vi "Pet Feeder.vi"() -> ()   [LabVIEW 2019, in "Pet Feeder.lvlib"]
uses:
  Pet Feeder.lvlib
  Types/app_event.ctl
  Types/state_machine_event.ctl
  Controls/Feeder Program.ctl
  Types/internal_state_data.ctl
  Types/state.ctl
panel:
  in  "clear last?":bool
  out "state":T1
  out "internal state data":T2 {"last dispense time" format="%<%H:%M:%S>t"; "clock time" format="%<%H:%M:%S>t"}
  in  "stop":bool
  in  "hopper level":i32=16
  out "hopper empty":bool
  out "hopper low":bool
  in  "set hopper":bool
  in  "set simulated time":bool
  in  "simulated time":string(combo)="1:00:00 PM"
  out "timer (s)":dbl format="%1.1g"
  out "remaining servings":i32(slide) scale=0.0..100.0
  in  "decrement servings":bool
  in  "increment servings":bool
  in  "program mode":string(combo)="none"
  in  "decrement minute":bool
  in  "increment minute":bool
  in  "decrement hour":bool
  in  "increment hour":bool
  out "current time":string
  out "schedule":T3[](array[typedef])
  in  "dispense serving":bool
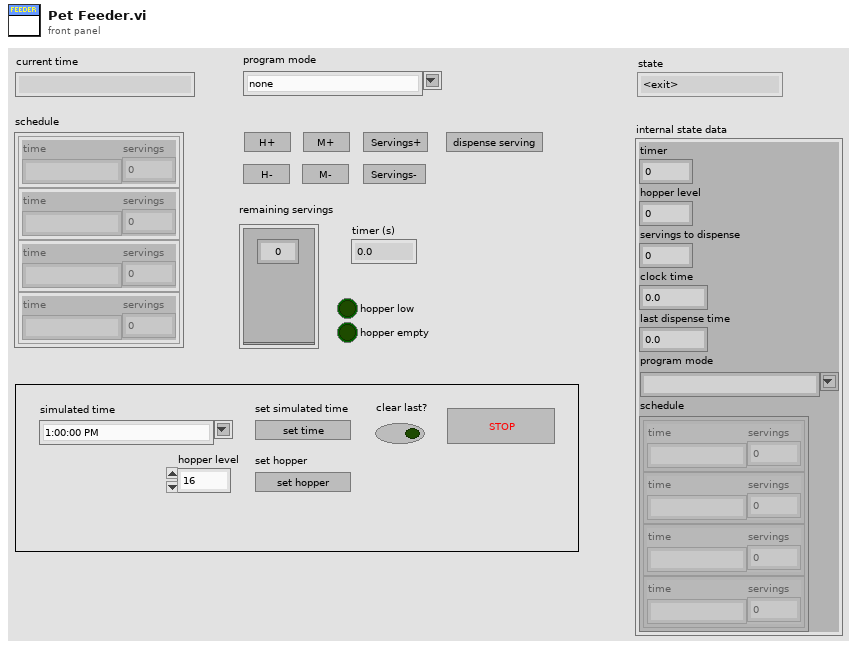
[diagram p1: front panel]
types:
  T1 = typedef "Pet Feeder.lvlib/state.ctl" = enum16{"<exit>", "<entry>", "idle", "dispensing"}
  T2 = typedef "Pet Feeder.lvlib/internal_state_data.ctl" = cluster{"timer":dbl, "hopper level":i32, "servings to dispense":i32, "clock time":dbl, "last dispense time":dbl, "program mode":string, "schedule":T3[]}
  T3 = typedef "Pet Feeder.lvlib/Feeder Program.ctl" = cluster{"time":string, "servings":i32}
  T4 = typedef "Pet Feeder.lvlib/state_machine_event.ctl" = cluster{"event":enum16{"button press", "timeout"}, "data":string}
  T5 = typedef "Pet Feeder.lvlib/app_event.ctl" = enum16{"Initialize", "Shutdown", "Exit"}
  T6 = cluster{"event":enum16{"button press", "timeout"}, "data":string}
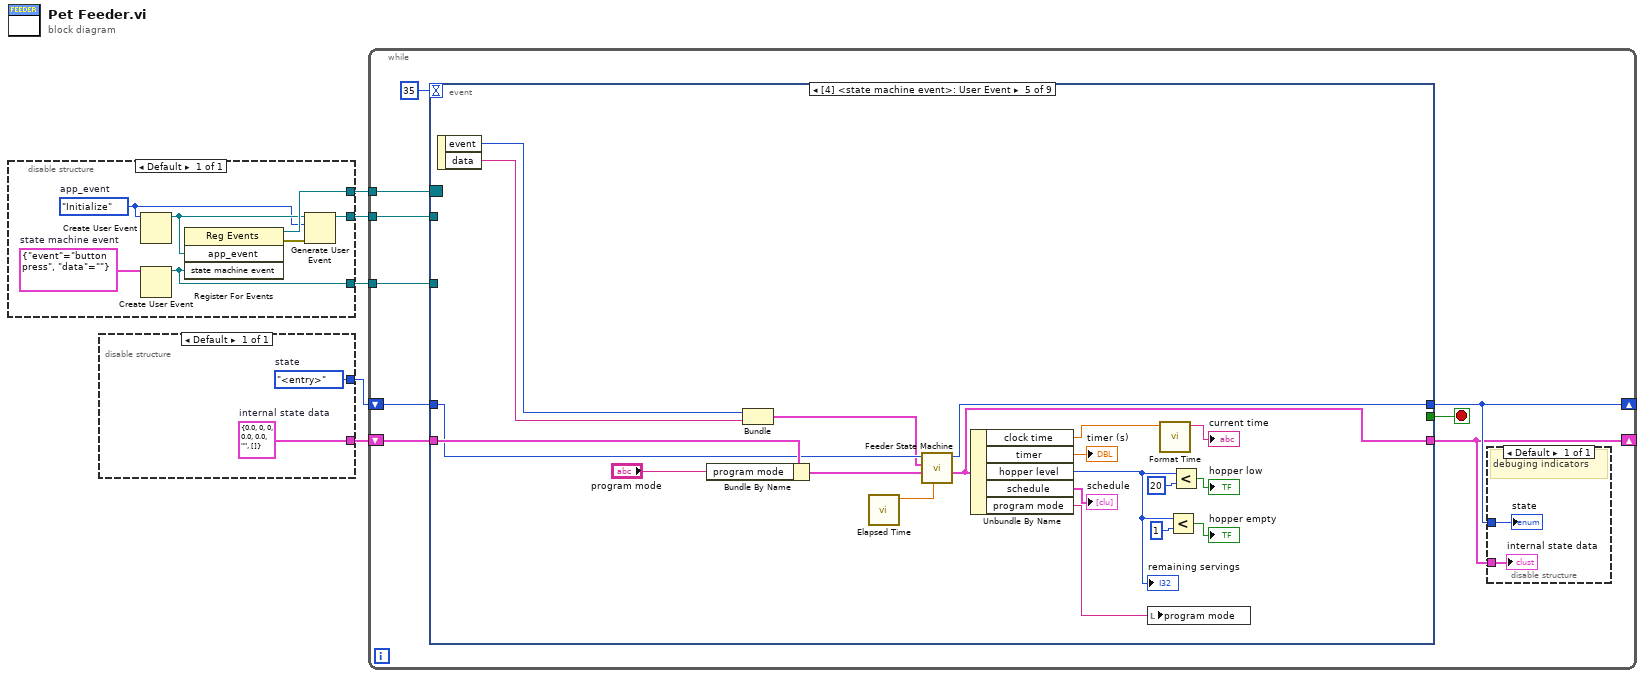
[diagram p0: block diagram]
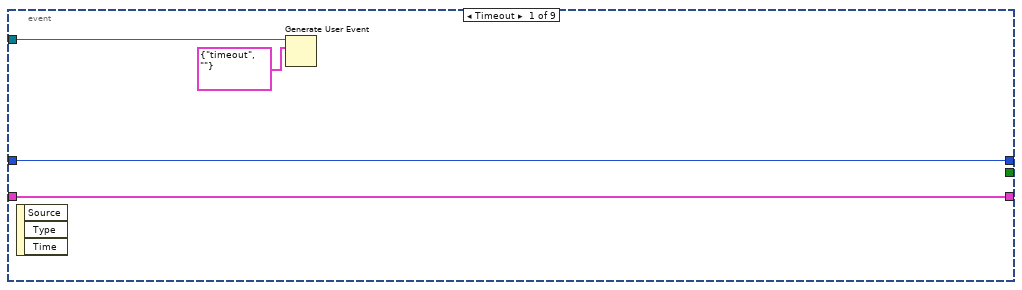
[diagram p2: hidden frame]
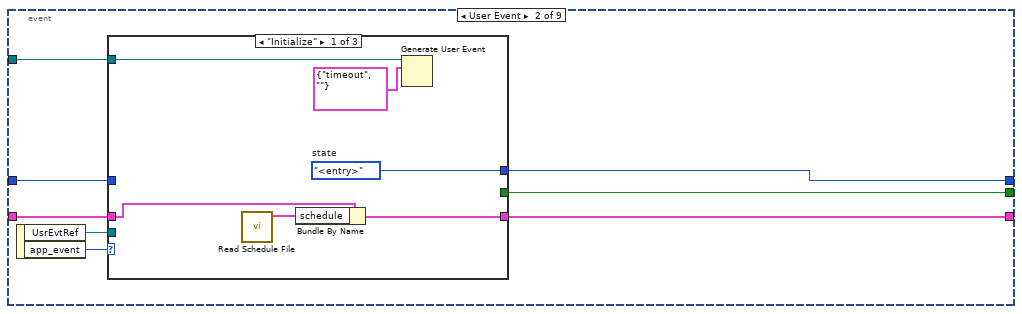
[diagram p3: hidden frame]
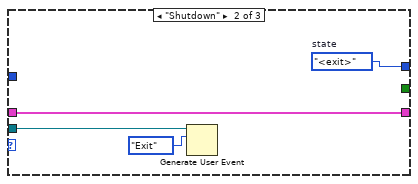
[diagram p4: hidden frame]
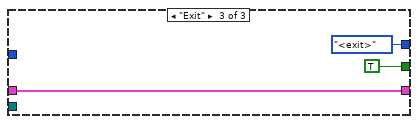
[diagram p5: hidden frame]
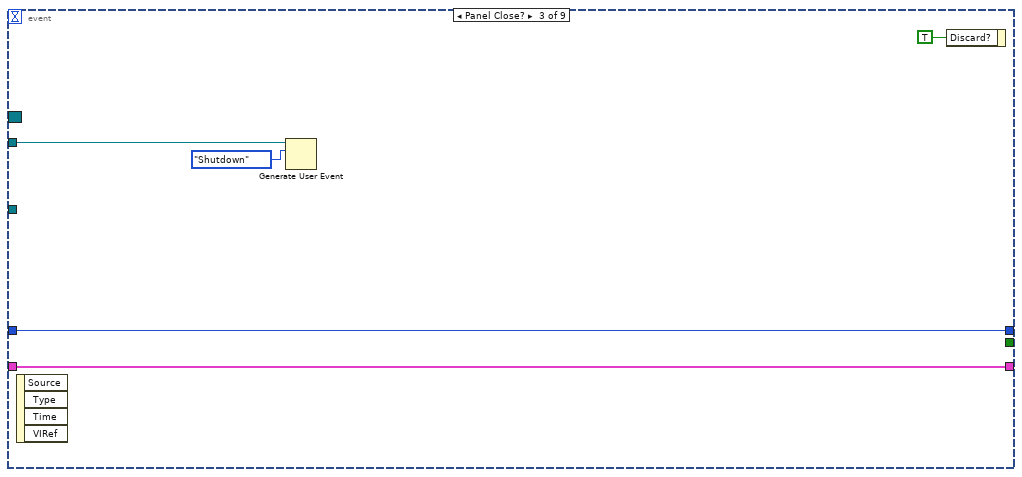
[diagram p6: hidden frame]
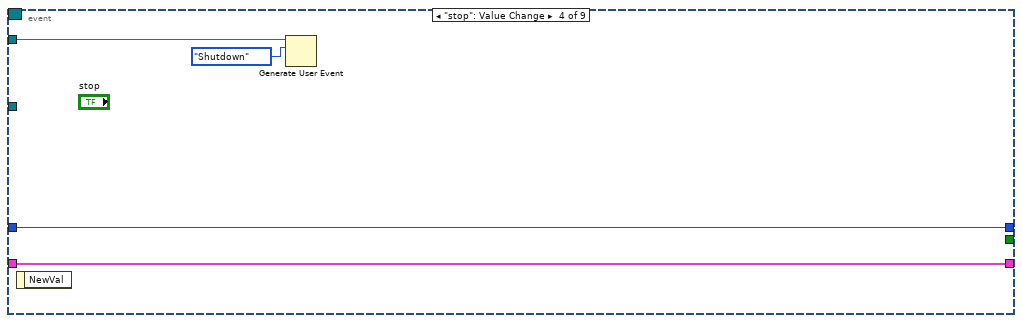
[diagram p7: hidden frame]
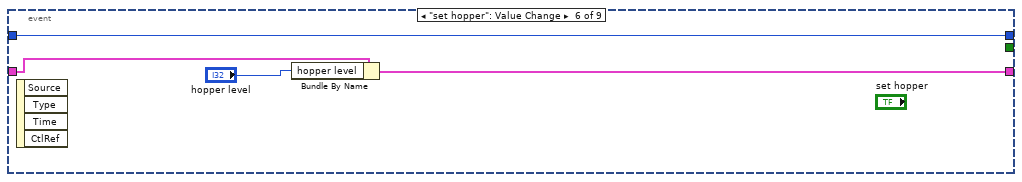
[diagram p8: hidden frame]
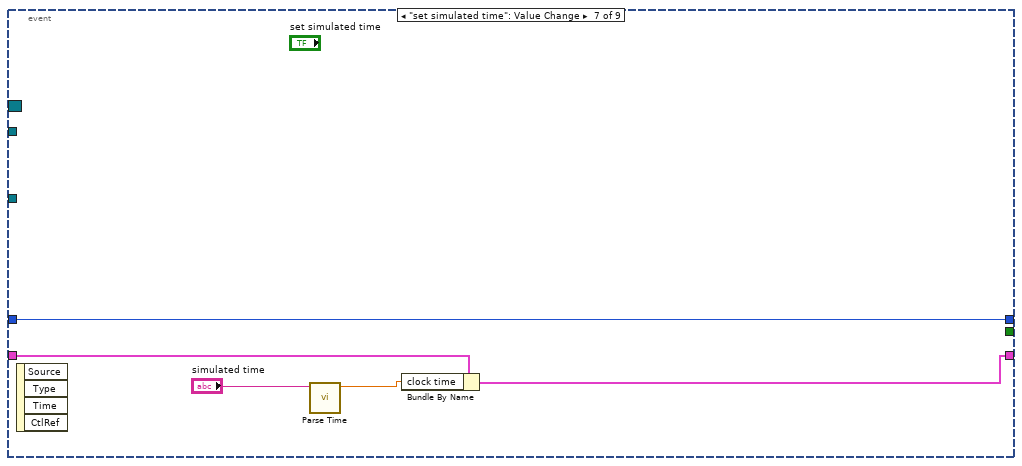
[diagram p9: hidden frame]
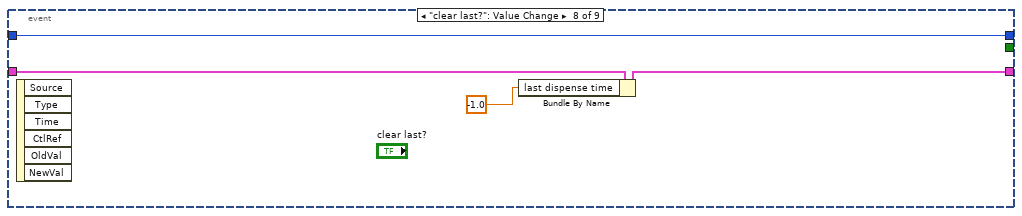
[diagram p10: hidden frame]
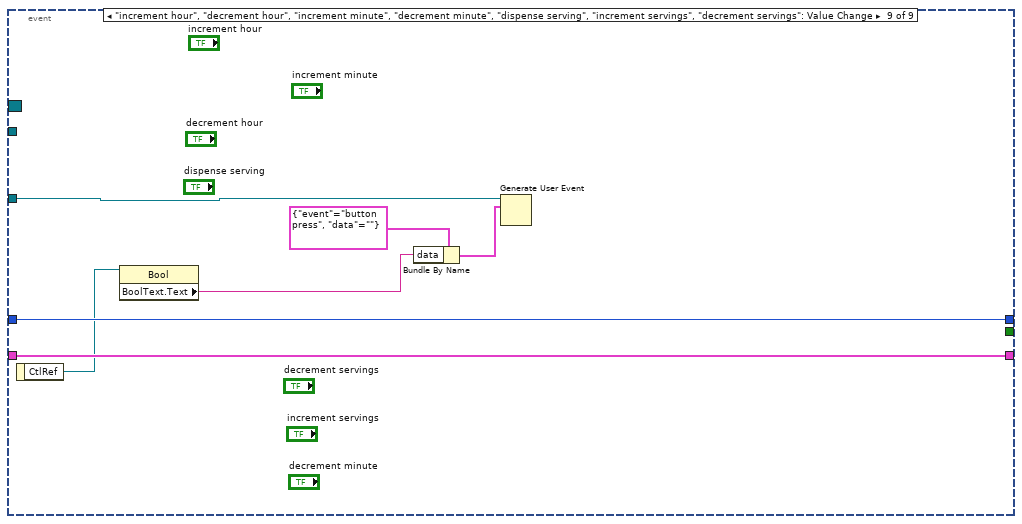
[diagram p11: hidden frame]
diagram:
  n1 = disable-structure shown="Default" {
    disable-tunnel: [w12] -> w5
    disable-tunnel: [w7] -> w4
    disable-tunnel: [w6] -> w3
    frame Enabled {
      w11 = T4 {"event"=enum."button press", "data"=""}  # state machine event
      w8 = app_event."Initialize"  # app_event
      n2 = Create User Event(user event datatype=w8) -> (user event=w10:refnum<user-event>)  [unwired: 1 in, 1 out]
      n3 = Create User Event(user event datatype=w11) -> (user event=w6:refnum<user-event>)  [unwired: 1 in, 1 out]
      n4 = register-events(w10, w6) -> (reference out=w12:refnum<event-registration>, error out=w9:errorcluster)  [unwired: 2 in]
      n5 = Generate User Event(user event=w10, event data cluster=w8, error in=w9) -> (user event out=w7:refnum<user-event>)  [unwired: 1 in, 1 out]
    }
  }
  n6 = disable-structure shown="Default" {
    disable-tunnel: [w14] -> w2
    disable-tunnel: [w13] -> w1
    frame Enabled {
      w14 = state."<entry>"  # state
      w13 = T2 {"timer"=0.0, "hopper level"=0, "servings to dispense"=0, "clock time"=0.0, "last dispense time"=0.0, "program mode"="", "schedule"=[]}  # internal state data
    }
  }
  n7 = while {
    tunnel: w5 -> [w23]
    tunnel: w4 -> [w15]
    tunnel: w3 -> [w18]
    shift-right: [w21] -> _
    shift-left: w2 -> [w22]
    shift-right: [w20] -> _
    shift-left: w1 -> [w19]
    stop <- w17 stop-if-true
    n8 = event shown="[4] <state machine event>: User Event" {
      selector: w23 -> [_ _ _ _ _ _ _ _ _]
      dyn-events: _ -> [_ _ _ _ _ _ _ _ _]
      timeout: 35 -> [_ _ _ _ _ _ _ _ _]
      tunnel: w22 -> [w29 w30 w55 w59 w75 w83 w88 w92 w99]
      tunnel: [w29 w31 w55 w59 w76 w83 w88 w92 w99] -> w21
      tunnel: [w28 w32 w54 w58 w69 w81 w86 w90 w98] -> w20
      tunnel: w19 -> [w28 w33 w54 w58 w77 w82 w87 w91 w98]
      tunnel: w18 -> [w27 w35 _ _ _ _ _ _ w96]
      tunnel: [_ w34 _ _ _ _ _ _ _] -> w17
      tunnel: w15 -> [_ _ w52 w57 _ _ _ _ _]
      event Timeout {
        n9 = event-data() -> ()  [unwired: 1 in, 3 out]
        n10 = Generate User Event(user event=w27, event data cluster=T4 {"event"=enum."timeout", "data"=""} ("event data")) -> ()  [unwired: 2 in, 2 out]
      }
      event User Event {
        n11 = event-data() -> ("UsrEvtRef"=w37:refnum<user-event>, "app_event"=w36:T5)  [unwired: 1 in]
        n12 = case shown="\"Initialize\"" w36 {
          tunnel: w37 -> [_ w47 _]
          tunnel: w35 -> [w43 _ _]
          tunnel: [_ _ TRUE] -> w34
          tunnel: [w40 w45 w49] -> w32
          tunnel: w33 -> [w41 w45 w49]
          tunnel: [w38 w44 state."<exit>" ("state")] -> w31
          tunnel: w30 -> [_ _ _]
          frame "Initialize" {
            w38 = state."<entry>"  # state
            n13 = call "Read Schedule File.vi"() -> ("meal schedule"=w39:T3[])  [unwired: 10 in, 1 out]
            n14 = Bundle By Name(cluster=w41, "schedule"=w39) -> (w40:T2)
            n15 = Generate User Event(user event=w43, event data cluster=T4 {"event"=enum."timeout", "data"=""} ("event data")) -> ()  [unwired: 2 in, 2 out]
          }
          frame "Shutdown" {
            w44 = state."<exit>"  # state
            n16 = Generate User Event(user event=w47, event data cluster=app_event."Exit" ("event data")) -> ()  [unwired: 2 in, 2 out]
          }
          frame "Exit" {
          }
        }
      }
      event Panel Close? {
        n17 = event-data() -> ()  [unwired: 1 in, 4 out]
        n18 = Generate User Event(user event=w52, event data cluster=app_event."Shutdown" ("event data")) -> ()  [unwired: 2 in, 2 out]
        n19 = event-data("Discard?"=TRUE) -> ()  [unwired: 1 in, 1 out]
      }
      event "stop": Value Change {
        n20 = event-data() -> ()  [unwired: 1 in, 1 out]
        n21 = Generate User Event(user event=w57, event data cluster=app_event."Shutdown" ("event data")) -> ()  [unwired: 2 in, 2 out]
      }
      event User Event {
        n22 = event-data() -> ("event"=w79:enum16{"button press", "timeout"}, "data"=w78:string)  [unwired: 1 in]
        n23 = Bundle By Name(cluster=w77, "program mode"="program mode") -> (w67:T2)
        n24 = Bundle("event"=w79, "data"=w78) -> (w74:T6)  [unwired: 1 in]
        n25 = call "Elapsed Time.vi"() -> ("elapsed time (s)"=w73:dbl)  [unwired: 11 in]
        n26 = call "Feeder State Machine.vi"("elapsed time(s)"=w73, "state data in"=w67, "state machine event"=w74, "state in"=w75) -> ("state data out"=w69:T2, "state out"=w76:T1)  [unwired: 6 in]
        n27 = Unbundle By Name(w69) -> ("clock time"=w71:dbl, "timer"=→"timer (s)":dbl, "hopper level"=w61:i32, "schedule"=→"schedule":T3[], "program mode"=w65:string)
        "remaining servings" <- w61
        n28 = local write "program mode"(w65) -> ()
        n29 = call "Format Time.vi"("time (HH:MM:SS)"=w71) -> ("time string"=→"current time":string)  [unwired: 10 in]
        n30 = Less?(x=w61, y=1) -> (x < y?=→"hopper empty":bool)
        n31 = Less?(x=w61, y=20) -> (x < y?=→"hopper low":bool)
      }
      event "set hopper": Value Change {
        n32 = event-data() -> ()  [unwired: 1 in, 4 out]
        n33 = Bundle By Name(cluster=w82, "hopper level"="hopper level") -> (w81:T2)
      }
      event "set simulated time": Value Change {
        n34 = event-data() -> ()  [unwired: 1 in, 4 out]
        n35 = call "Parse Time.vi"("parse time"="simulated time") -> ("time (HH:MM:SS)"=w84:dbl)  [unwired: 10 in]
        n36 = Bundle By Name(cluster=w87, "clock time"=w84) -> (w86:T2)
      }
      event "clear last?": Value Change {
        n37 = event-data() -> ()  [unwired: 1 in, 6 out]
        n38 = Bundle By Name(cluster=w91, "last dispense time"=-1.0) -> (w90:T2)
      }
      event "increment hour", "decrement hour", "increment minute", "decrement minute", "dispense serving", "increment servings", "decrement servings": Value Change {
        n39 = event-data() -> ("CtlRef"=w97:refnum<vi>)  [unwired: 1 in]
        n40 = property class="Bool"(reference=w97) -> ("BoolText.Text"=w93:string)  [unwired: 1 in, 2 out]
        n41 = Bundle By Name(cluster=T4 {"event"=enum."button press", "data"=""} ("event data"), "data"=w93) -> (w94:T4)
        n42 = Generate User Event(user event=w96, event data cluster=w94) -> ()  [unwired: 2 in, 2 out]
      }
    }
    n43 = disable-structure shown="Default" {
      disable-tunnel: w21 -> [w25]
      disable-tunnel: w20 -> [w24]
      frame Enabled {
        # "debuging indicators"
        "internal state data" <- w24
        "state" <- w25
      }
    }
  }
